vi "CRYAnalyt.vi"(4 "Input":dbl[](array[numeric])=[0.0, 0.0, 0.0, 0.0, 0.0, 1.0, 0.0, 0.0, 0.0, 0.0, 0.0] format="%.2f") -> (0 "Magn":dbl[](array[numeric])=[0.12716412468699562, 0.0, 0.21211070832577886, 0.0, 0.6365878141136418, 1.0, 0.6365878141136421, 0.0, 0.21211070832577902, 0.0, 0.12716412468699528] format="%.2f", 1 "Imag":dbl[](array[numeric])=[-0.12716412468699562, 0.0, -0.21211070832577886, 0.0, -0.6365878141136418, 0.0, 0.6365878141136421, 0.0, 0.21211070832577902, 0.0, 0.12716412468699528] format="%.2f", 2 "Real":dbl[](array[numeric])=[0.0, 0.0, 0.0, 0.0, 0.0, 1.0, 0.0, 0.0, 0.0, 0.0, 0.0] format="%.2f")   [LabVIEW 2013]
uses:
  <vilib>/Analysis/4window.llb/Flat Top Window (DBL).vi
  <vilib>/Analysis/2dsp.llb/1D Convolution (DBL).vi
  <vilib>/Analysis/4window.llb/AllCosWindow (DBL).vi
  <vilib>/Analysis/NI_AALBase.lvlib
  <vilib>/Analysis/NI_AALPro.lvlib
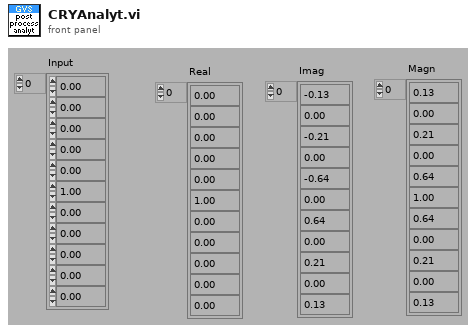
[diagram p1: front panel]
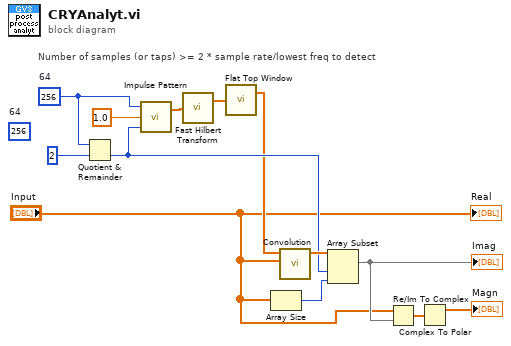
[diagram p0: block diagram]
diagram:
  (unwired) 256  # 64
  w11 = 256  # 64
  # "Number of samples (or taps) >= 2 * sample rate/lowest freq to detect"
  n1 = Quotient & Remainder(x=w11, y=2) -> (floor(x/y)=w6:i32)  [unwired: 1 out]
  n2 = call <vilib>:"Impulse Pattern.vi"("delay"=w6, "amplitude"=1.0, "samples"=w11) -> ("Impulse Pattern"=w4:dbl[])  [unwired: 1 out]
  n3 = call <vilib>:"Fast Hilbert Transform.vi"("X"=w4) -> ("Hilbert{X}"=w5:dbl[])  [unwired: 1 out]
  n4 = call-poly <vilib>:"Flat Top Window.vi"("X"=w5) -> ("Windowed X"=w3:dbl[])  [unwired: 1 out]
  n5 = Array Size(array="Input") -> (size(s)=w7:i32)
  n6 = call-poly <vilib>:"Convolution.vi"("Y"="Input", "X"=w3) -> ("X * Y"=w9:dbl[])  [unwired: 1 in, 8 out]
  n7 = Array Subset(array=w9, index=w6, length=w7) -> (w8:dbl[])
  "Imag" <- w8
  n8 = Re/Im To Complex(1:w8, 2:"Input") -> (0:w12:cdb[])
  n9 = Complex To Polar(r * e^(i*theta)=w12) -> (r=→"Magn":dbl[])  [unwired: 1 out]
  "Real" <- "Input"
